vi "ChartBar.vi"(11 "Array":u8[](array[numeric])) -> (3 "XY Graph":cluster{i32[], "Array":u8[]}(graph))   [LabVIEW 2014]
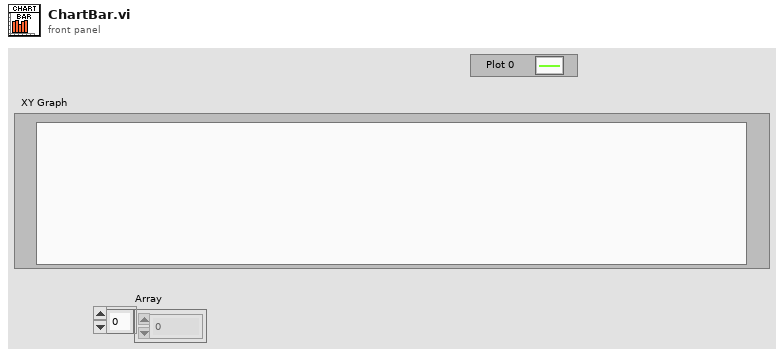
[diagram p1: front panel]
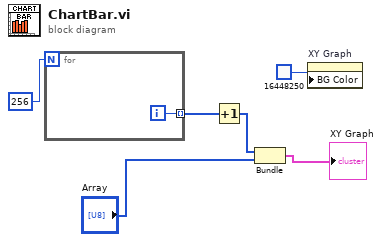
[diagram p0: block diagram]
diagram:
  n1 = for {
    N: 256 -> [_]
    tunnel: [w7] -> w4 mode=indexing
    i -> [w7]
  }
  n2 = Increment(x=w4) -> (x+1=w3:i32[])
  n3 = Bundle(w3, "Array"="Array") -> (→"XY Graph":cluster{i32[], "Array":u8[]})  [unwired: 1 in]
  n4 = property on="XY Graph" class="XYGraph (strict)"("BG Color"=u32 16448250) -> ()  [unwired: 2 in, 2 out]
